vi "Call Actor-Run.vi"(8 "error in (no error)":errorcluster, 9 "Front Panel State":T1, 10 "API-Requests":T2, 11 "Actor in":refnum<class "Actor.lvclass">) -> (0 "error out":errorcluster, 3 "Actor out":refnum<class "Actor.lvclass">)   [LabVIEW 2018, in "Scripting.lvlib" / "Actor.lvlib" / "Actor.lvclass"]
uses:
  Actor.lvclass
  API-Requests.ctl
  Launched.ctl
  Stop.ctl
  Get State.ctl
  State.ctl
  Front-Panel State.ctl
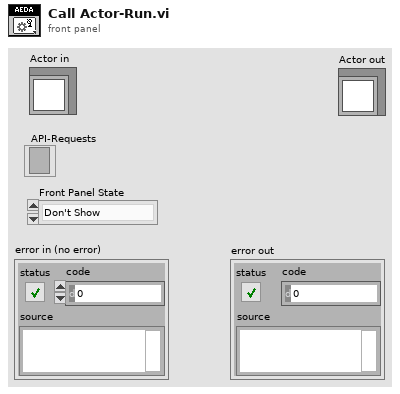
[diagram p1: front panel]
types:
  T1 = typedef "Scripting.lvlib/Actor.lvlib/Actor.lvclass/Front-Panel State.ctl" = enum16{"Don't Show", "Show"}
  T2 = typedef "Scripting.lvlib/Actor.lvlib/Actor.lvclass/API-Requests.ctl" = refnum<event-registration>
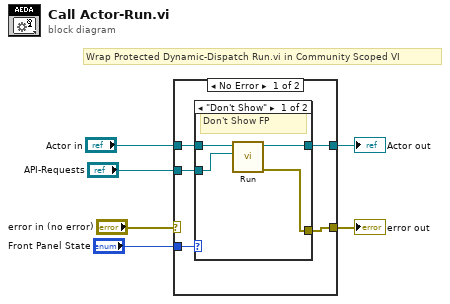
[diagram p0: block diagram]
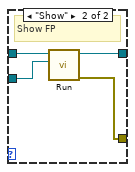
[diagram p2: hidden frame]
diagram:
  # "Wrap Protected Dynamic-Dispatch Run.vi in Community Scoped VI"
  n1 = case shown="No Error" "error in (no error)" {
    selector: "error in (no error)" -> [_ w21]
    tunnel: "API-Requests" -> [w11 _]
    tunnel: [w10 w21] -> w5
    tunnel: [w9 w20] -> w4
    tunnel: "Actor in" -> [w8 w20]
    tunnel: "Front Panel State" -> [w7 _]
    frame No Error {
      n2 = case shown="\"Don't Show\"" w7 {
        tunnel: w8 -> [w15 w19]
        tunnel: [w14 w18] -> w10
        tunnel: [w13 w17] -> w9
        tunnel: w11 -> [w12 w16]
        frame "Don't Show" {
          # "Don't Show FP"
          n3 = call-dynamic "Run.vi"("API-Requests"=w12, "Actor in"=w15) -> ("error out"=w14:errorcluster, "Actor out"=w13:refnum<class "Actor.lvclass">)  [unwired: 8 in]
        }
        frame "Show" {
          # "Show FP"
          n4 = call-dynamic "Run.vi"("API-Requests"=w16, "Actor in"=w19) -> ("error out"=w18:errorcluster, "Actor out"=w17:refnum<class "Actor.lvclass">)  [unwired: 8 in]
        }
      }
    }
    frame Error {
    }
  }
  "error out" <- w5
  "Actor out" <- w4
